vi "Edge Detection with Wavelets.vi"() -> ()   [LabVIEW 2023]
doc: "This example shows the application of the wavelet transforms in detecting image edges.\n\nConventional edge detection methods process an image at a single resolution and return a binary edge map. The wavelet transform-based method processes an image at multiple levels of resolution and returns a series of grey-level edge maps at different resolutions. You can obtain the global profile of the image in a low-resolution edge map and the detailed texture of the image in a high-resolution edge map.\n\nThis example uses the WA Multiscale Edge Detection VI to detect the edges of an image.\n\n<b>Instructions:</b>\n1) Run this VI.\n2) Increase the value of <b>Level</b> to observe coarser edges.\n3) Increase the value of <b>Threshold Ratio</b> to skip the edges in darker areas."
uses:
  Images/_Images.ctl
  <vilib>/addons/_Advanced Signal Processing/NI_AdvSigProcWA.lvlib
panel:
  out "Phase":T1(plugin-control)
  out "Magnitude":T1(plugin-control)
  in  "Image":T2=enum."Balls2"
  in  "wavelet":u16(ring)=20 items=["db02"=0, "db03"=1, "db04"=2, "db05"=3, "db06"=4, "db07"=5, "db08"=6, "db09"=7, "db10"=8, "db11"=9, "db12"=10, "db13"=11, "db14"=12, "Haar"=13, "bior1_3"=14, "bior1_5"=15, "bior2_2"=16, "bior2_4"=17, "bior2_6"=18, "bior2_8"=19, "bior3_1"=20, "bior3_3"=21, "bior3_5"=22, "bior3_7"=23, "bior3_9"=24, "bior4_4 (FBI)"=25, "bior5_5"=38, "bior6_8"=39, "coif1"=26, "coif2"=27, "coif3"=28, "coif4"=29, "coif5"=30, "sym2"=31, "sym3"=32, "sym4"=33, "sym5"=34, "sym6"=35, "sym7"=36, "sym8"=37]
  out "Edges":T1(plugin-control)
  out "Source Image":T1(plugin-control)
  out "Edge":i16[][](graph)
  in  "Level":i32=1 min=1 max=8
  in  "Threshold ratio":dbl=0.1 min=0.0001 max=1.0 step=0.1
  # "Edges detection using Wavelets"
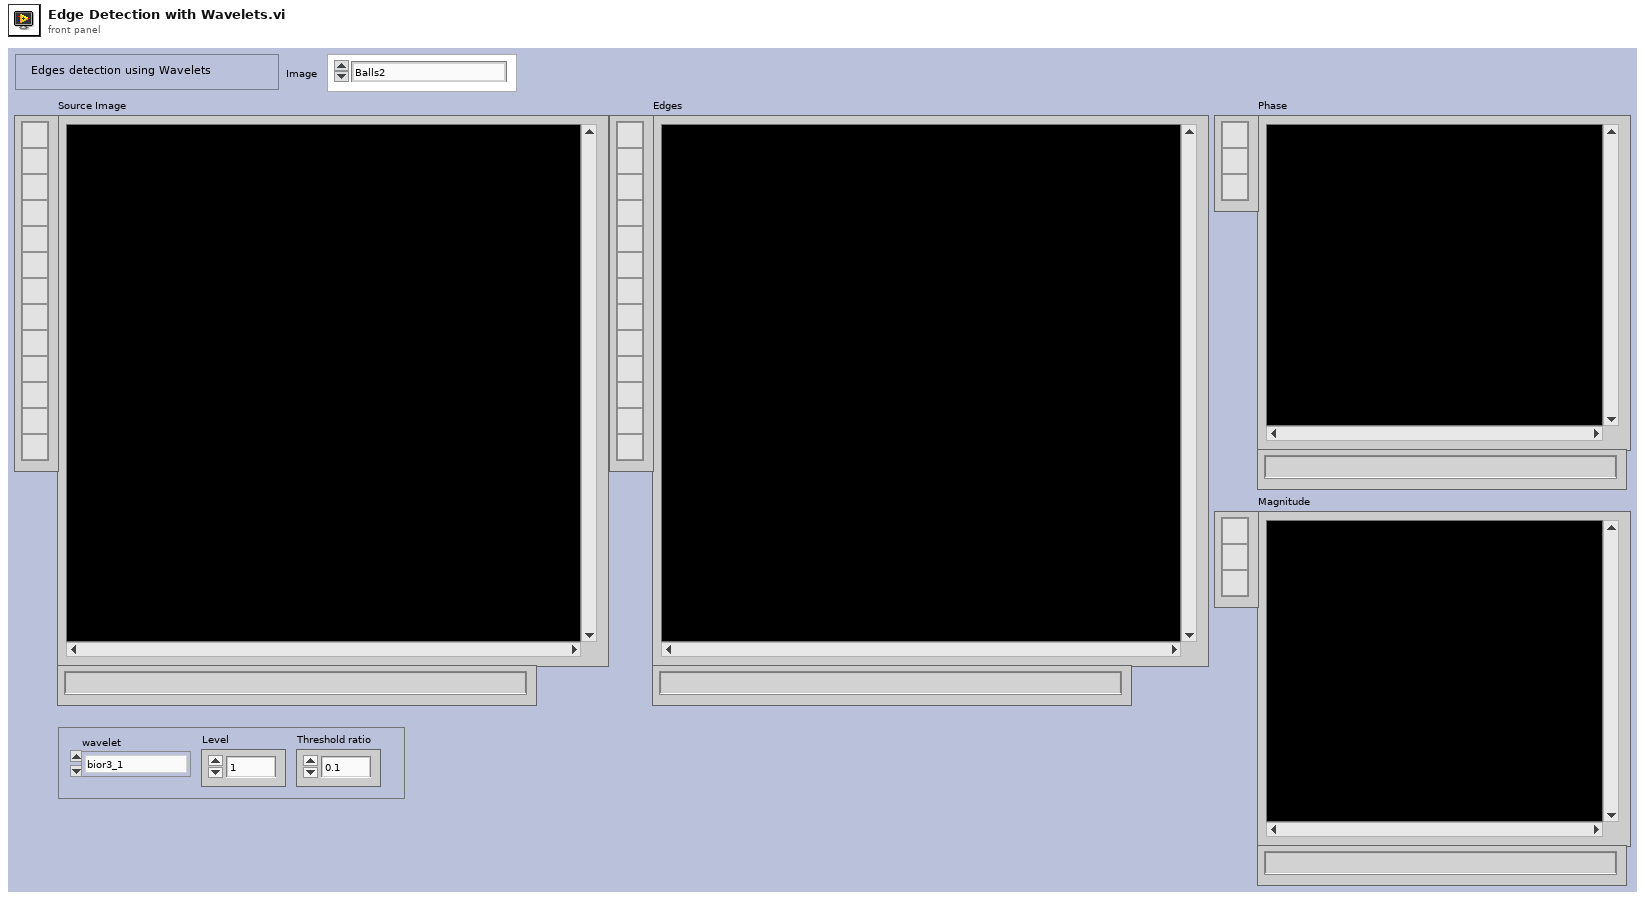
[diagram p1: front panel]
types:
  T1 = typedef "IMAQ Image.ctl" = refnum<image>
  T2 = typedef "_Images.ctl" = enum16{"Ostern2023", "Balls2", "Battery1", "Battery2", "Connector1", "Subwoofer1", "Subwoofer2", "Subwoofer3", "Subwoofer4", "Hase1", "Lamp1", "Lamp2", "Mouse1", "PhotoLens1", "Po1", "PowerSupply1", "Router", "--- Step Wedges ---", "Stepwedge1", "Stepwedge2", "Stepwedge3", "--- Fusion ---", "Fusion160kV", "Fusion2-120kV", "Fusion2-320kV", "Fusion300kV", "FusionPart1-120kV", "FusionPart1-180kV", "--- PART 01 ---", "Part1", "Part2", "Part3", "Part4", "Part5", "Part6", "Part7", "Part8", "--- Different Integrations ---", "Step2737-02Int", "Step2737-04Int", "Step2737-08Int", "Step2737-16Int", "Step2737-32Int", "Step2737-64Int"}
  T3 = typedef "Image Type" = u32
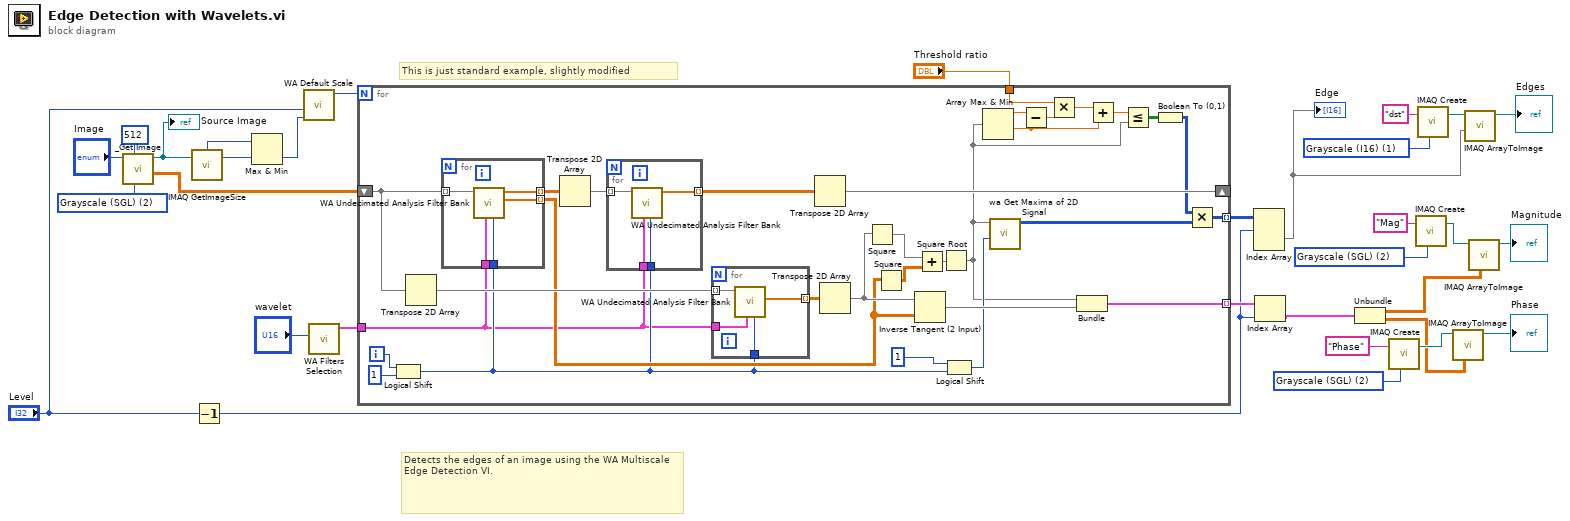
[diagram p0: block diagram]
diagram:
  w12 = T3 2 items=["Grayscale (U8)", "Grayscale (I16)", "Grayscale (SGL)", "Complex (CSG)", "RGB (U32)", "HSL (U32)", "RGB (U64)", "Grayscale (U16)"] ("Image Type")
  w13 = T3 2 items=["Grayscale (U8)", "Grayscale (I16)", "Grayscale (SGL)", "Complex (CSG)", "RGB (U32)", "HSL (U32)", "RGB (U64)", "Grayscale (U16)"] ("Image Type")
  w24 = T3 1 items=["Grayscale (U8)", "Grayscale (I16)", "Grayscale (SGL)", "Complex (CSG)", "RGB (U32)", "HSL (U32)", "RGB (U64)", "Grayscale (U16)"] ("Image Type")
  w26 = T3 2 items=["Grayscale (U8)", "Grayscale (I16)", "Grayscale (SGL)", "Complex (CSG)", "RGB (U32)", "HSL (U32)", "RGB (U64)", "Grayscale (U16)"] ("Image Type (U16)")
  # "This is just standard example, slightly modified"
  # "Detects the edges of an image using the WA Multiscale Edge Detection VI."
  n1 = call "_Get Image.vi"("Image Type (U16)"=w26, "XY Resolution"=512, "Image"="Image") -> ("Image Pixels (Float)"=w25:dbl[][], "Image Out"=w4:T1)  [unwired: 5 in, 2 out]
  "Source Image" <- w4
  n2 = call "IMAQ GetImageSize"("Image"=w4) -> ("Y Resolution"=w2:i32, "X Resolution"=w3:i32)  [unwired: 3 in, 1 out]
  n3 = Decrement(x="Level") -> (x-1=w16:i32)
  n4 = Max & Min(x=w3, y=w2) -> (min(x,y)=w1:i32)  [unwired: 1 out]
  n5 = call <vilib>:"WA Default Scale.vi"("signal length"=w1, "level in"="Level") -> ("level out"=w30:i32)  [unwired: 1 in, 4 out]
  n6 = call <vilib>:"WA Filters Selection.vi"("wavelet"="wavelet") -> ("analysis filters"=w29:cluster{"lowpass":dbl[], "highpass":dbl[]})  [unwired: 2 in, 8 out]
  n7 = for {
    N: w30 -> [_]
    shift-right: [w60] -> _
    shift-left: w25 -> [w57]
    tunnel: [w51] -> w17 mode=indexing
    tunnel: w29 -> [w43]
    tunnel: "Threshold ratio" -> [w36]
    tunnel: [w33] -> w20 mode=indexing
    i -> [w48]
    n8 = Logical Shift(y=w48, x=1) -> (x << y=w45:i32)
    n9 = Transpose 2D Array(2D array=w57) -> (transposed array=w59:dbl[][])
    n10 = for {
      tunnel: w57 -> [w76] mode=indexing
      tunnel: [w75] -> w49 mode=indexing
      tunnel: [w74] -> w63 mode=indexing
      tunnel: w45 -> [w73]
      tunnel: w43 -> [w72]
      n11 = call <vilib>:"WA Undecimated Analysis Filter Bank.vi"("factor"=w73, "analysis filters"=w72, "X"=w76) -> ("Detail Coeffs"=w75:dbl[], "Apprx Coeffs"=w74:dbl[])  [unwired: 2 in, 5 out]
    }
    n12 = Transpose 2D Array(2D array=w63) -> (transposed array=w62:dbl[][])
    n13 = for {
      tunnel: w62 -> [w71] mode=indexing
      tunnel: [w70] -> w61 mode=indexing
      tunnel: w45 -> [w69]
      tunnel: w43 -> [w68]
      n14 = call <vilib>:"WA Undecimated Analysis Filter Bank.vi"("factor"=w69, "analysis filters"=w68, "X"=w71) -> ("Apprx Coeffs"=w70:dbl[])  [unwired: 2 in, 6 out]
    }
    n15 = for {
      tunnel: w59 -> [w67] mode=indexing
      tunnel: [w66] -> w58 mode=indexing
      tunnel: w45 -> [w65]
      tunnel: w43 -> [w64]
      n16 = call <vilib>:"WA Undecimated Analysis Filter Bank.vi"("factor"=w65, "analysis filters"=w64, "X"=w67) -> ("Detail Coeffs"=w66:dbl[])  [unwired: 2 in, 6 out]
    }
    n17 = Transpose 2D Array(2D array=w61) -> (transposed array=w60:dbl[][])
    n18 = Transpose 2D Array(2D array=w58) -> (transposed array=w50:dbl[][])
    n19 = Square(x=w50) -> (x^2=w55:dbl[][])
    n20 = Square(x=w49) -> (x^2=w56:dbl[][])
    n21 = Inverse Tangent (2 Input)(1:w49, 2:w50) -> (0:w52:dbl[][])
    n22 = Add(x=w55, y=w56) -> (x+y=w54:dbl[][])
    n23 = Square Root(x=w54) -> (sqrt(x)=w35:dbl[][])
    n24 = Logical Shift(y=1, x=w45) -> (x << y=w46:i32)
    n25 = Array Max & Min(array=w35) -> (max value=w38:dbl, min value=w40:dbl)  [unwired: 2 out]
    n26 = call <vilib>:"wa Get Maxima of 2D Signal.vi"("range"=w46, "Image"=w35) -> ("Edge"=w53:i16[][])  [unwired: 9 out]
    n27 = Subtract(x=w38, y=w40) -> (x-y=w39:dbl)
    n28 = Multiply(x=w36, y=w39) -> (x*y=w41:dbl)
    n29 = Bundle(w35, w52) -> (w51:cluster{dbl[][], dbl[][]})  [unwired: 1 out]
    n30 = Add(x=w41, y=w40) -> (x+y=w42:dbl)
    n31 = Less Or Equal?(x=w42, y=w35) -> (x <= y?=w37:bool[][])
    n32 = Boolean To (0,1)(Boolean=w37) -> (0, 1=w34:i16[][])
    n33 = Multiply(x=w34, y=w53) -> (x*y=w33:i16[][])
  }
  n34 = Index Array(array=w20, index (dim 0)=w16) -> (element=w19:i16[][])  [unwired: 2 in]
  "Edge" <- w19
  n35 = Index Array(array=w17, index=w16) -> (element=w15:cluster{dbl[][], dbl[][]})
  n36 = Unbundle(w15) -> (w9:dbl[][], w7:dbl[][])
  n37 = call "IMAQ Create"("Image Name"="Phase", "Image Type"=w12) -> ("New Image"=w8:T1)  [unwired: 3 in, 1 out]
  n38 = call "IMAQ Create"("Image Name"="Mag", "Image Type"=w13) -> ("New Image"=w10:T1)  [unwired: 3 in, 1 out]
  n39 = call "IMAQ Create"("Image Name"="dst", "Image Type"=w24) -> ("New Image"=w22:T1)  [unwired: 3 in, 1 out]
  n40 = call "IMAQ ArrayToImage"("Image Pixels (Float)"=w7, "Image"=w8) -> ("Image Out"=→"Phase":T1)  [unwired: 8 in, 1 out]
  n41 = call "IMAQ ArrayToImage"("Image Pixels (I16)"=w19, "Image"=w22) -> ("Image Out"=→"Edges":T1)  [unwired: 8 in, 1 out]
  n42 = call "IMAQ ArrayToImage"("Image Pixels (Float)"=w9, "Image"=w10) -> ("Image Out"=→"Magnitude":T1)  [unwired: 8 in, 1 out]
